vi "initialisationHWError.vi"(8 "error in (no error)":errorcluster, 11 "AtomChipHWC in":refnum<class "AtomChipHWC.lvclass">) -> (0 "error out":errorcluster, 3 "AtomChipHWC out":refnum<class "AtomChipHWC.lvclass">)   [LabVIEW 2009, in "Hardware.lvlib" / "HWControllers.lvlib" / "AtomChipHWC.lvclass"]
uses:
  AtomChipHWC.lvclass
  AtomChipHWC.lvclass/AtomChipHWC.ctl
  Channels/Digital/DigitalOutput.lvclass
  Channels/VoltOutput/AnalogOutput.lvclass
  Channels/DDSOutput/Generic/DDSOutput.lvclass
  Network Controllers/CameraNetworkController/CameraNetworkController.lvclass
  HWController.lvclass
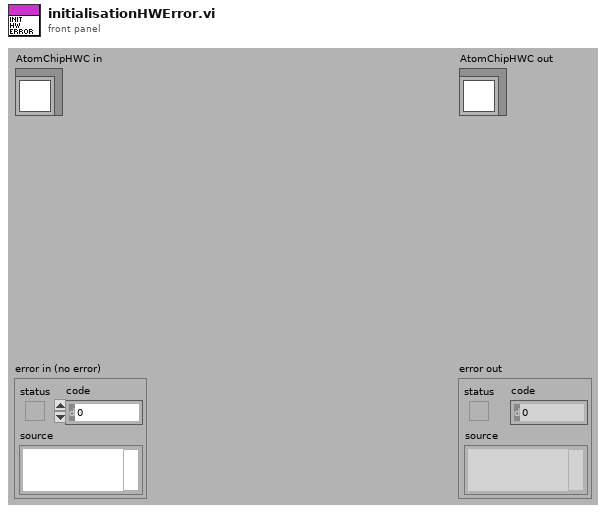
[diagram p1: front panel]
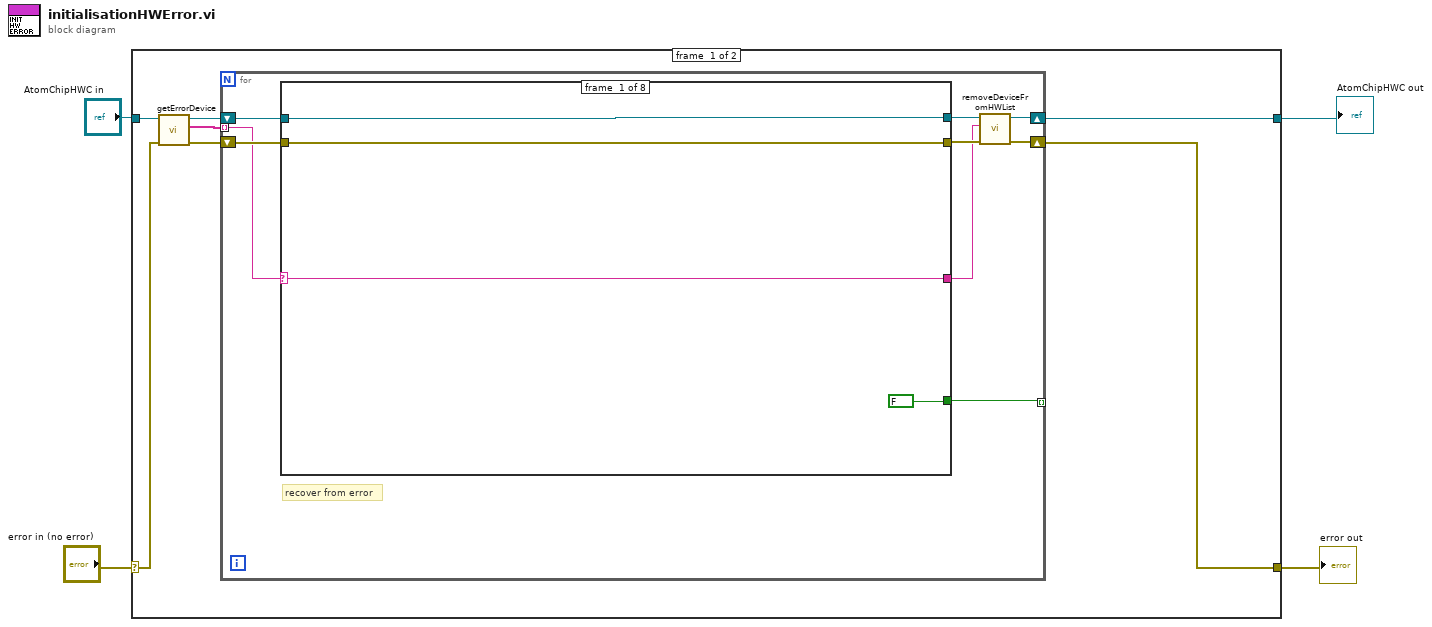
[diagram p0: block diagram]
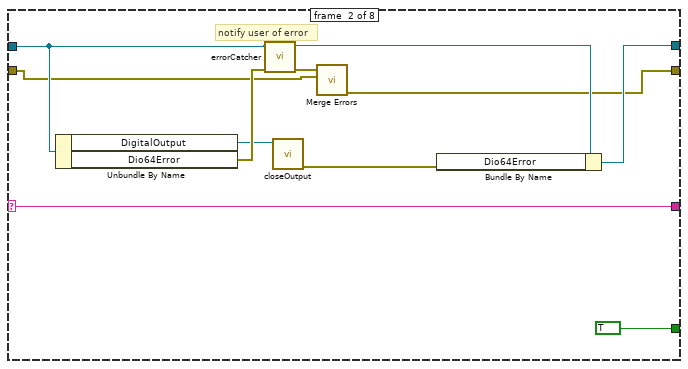
[diagram p2: hidden frame]
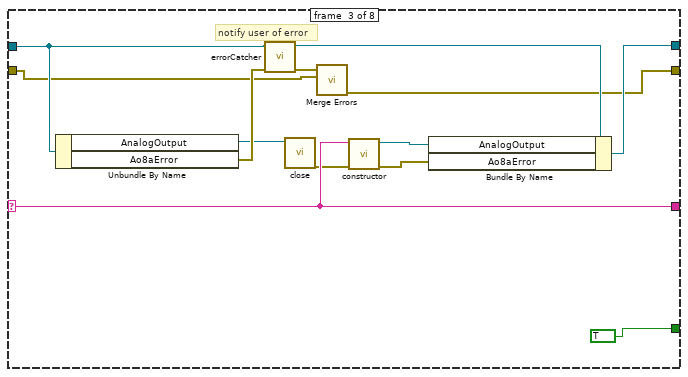
[diagram p3: hidden frame]
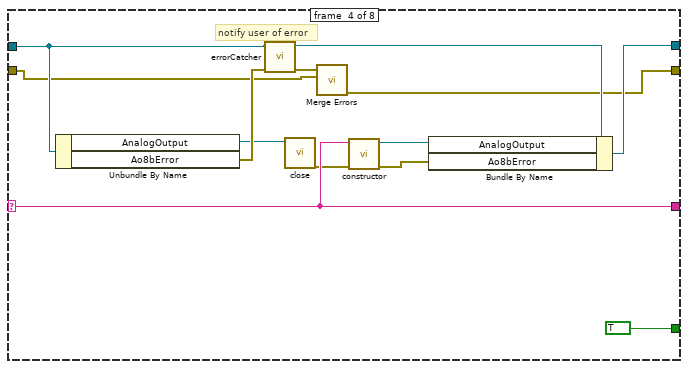
[diagram p4: hidden frame]
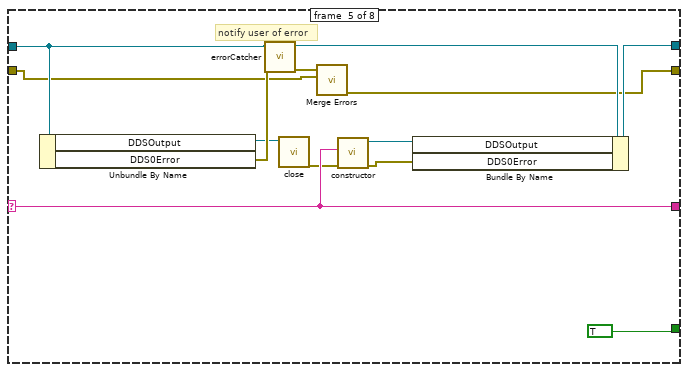
[diagram p5: hidden frame]
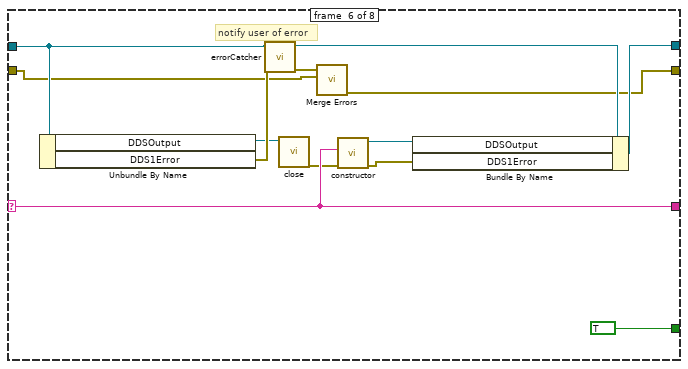
[diagram p6: hidden frame]
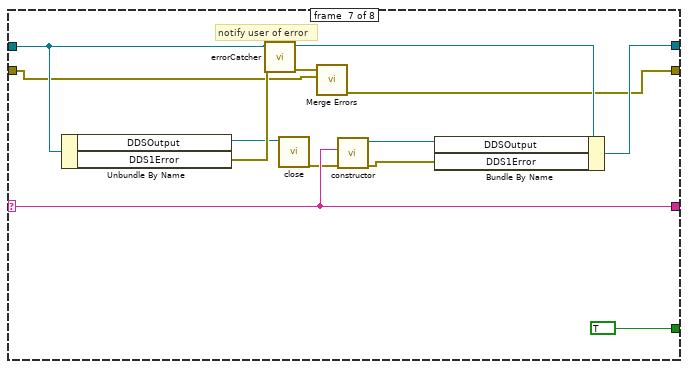
[diagram p7: hidden frame]
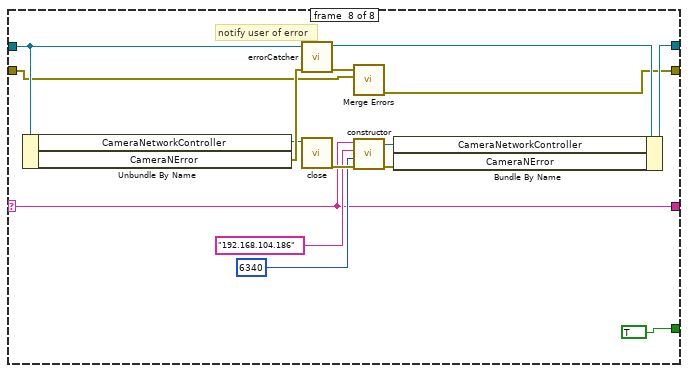
[diagram p8: hidden frame]
diagram:
  n1 = case shown="No Error" "error in (no error)" {
    selector: "error in (no error)" -> [w10 w116]
    tunnel: "AtomChipHWC in" -> [w11 w117]
    tunnel: [w6 w117] -> w2
    tunnel: [w5 w116] -> w1
    frame #0 {
      n2 = call "getErrorDevice.vi"("error in (no error)"=w10, "AtomChipHWC in"=w11) -> ("error out"=w7:errorcluster, "Devices"=w8:string[], "AtomChipHWC out"=w9:refnum<class "AtomChipHWC.lvclass">)  [unwired: 7 in]
      n3 = for {
        tunnel: w8 -> [w18] mode=indexing
        shift-right: [w14] -> w6
        shift-left: w9 -> [w20]
        shift-right: [w13] -> w5
        shift-left: w7 -> [w19]
        tunnel: [w12] -> _ mode=indexing
        # "recover from error"
        n4 = case shown="\"k3390\"" w18 {
          selector: w18 -> [w22 w28 w40 w53 w64 w77 w90 w102]
          tunnel: w20 -> [w24 w35 w48 w61 w74 w87 w100 w115]
          tunnel: [w24 w30 w43 w56 w69 w82 w95 w110] -> w17
          tunnel: [w23 w29 w42 w55 w68 w81 w94 w109] -> w16
          tunnel: w19 -> [w23 w31 w44 w57 w70 w83 w96 w111]
          tunnel: [w22 w28 w40 w53 w64 w77 w90 w102] -> w15
          tunnel: [FALSE TRUE TRUE TRUE TRUE TRUE TRUE TRUE] -> w12
          frame #0 {
          }
          frame #1 {
            # "notify user of error"
            n5 = Unbundle By Name(w35) -> ("DigitalOutput"=w26:refnum<class "DigitalOutput.lvclass">, "Dio64Error"=w33:errorcluster)
            n6 = call-dynamic "errorCatcher.vi"("error in (no error)"=w33, "HWController in"=w35) -> ("error out"=w32:errorcluster, "HWController out"=w34:refnum<class "AtomChipHWC.lvclass">)  [unwired: 8 in]
            n7 = call-dynamic "closeOutput.vi"("DigitalOutput in"=w26) -> ("error out"=w27:errorcluster)  [unwired: 10 in]
            n8 = call <vilib>:"Merge Errors.vi"("error in 2 (no error)"=w31, "error in 1 (no error)"=w32) -> ("error out"=w29:errorcluster)  [unwired: 5 in]
            n9 = Bundle By Name(cluster=w34, "Dio64Error"=w27) -> (w30:refnum<class "AtomChipHWC.lvclass">)
          }
          frame #2 {
            # "notify user of error"
            n10 = Unbundle By Name(w48) -> ("AnalogOutput"=w41:refnum<class "AnalogOutput.lvclass">, "Ao8aError"=w46:errorcluster)
            n11 = call-dynamic "errorCatcher.vi"("error in (no error)"=w46, "HWController in"=w48) -> ("error out"=w45:errorcluster, "HWController out"=w47:refnum<class "AtomChipHWC.lvclass">)  [unwired: 8 in]
            n12 = call-dynamic "close.vi"("AnalogOutput in"=w41) -> ("error out"=w39:errorcluster)  [unwired: 10 in]
            n13 = call <vilib>:"Merge Errors.vi"("error in 2 (no error)"=w44, "error in 1 (no error)"=w45) -> ("error out"=w42:errorcluster)  [unwired: 5 in]
            n14 = call "constructor.vi"("error in (no error)"=w39, "deviceName"=w40) -> ("error out"=w37:errorcluster, "AnalogOutput out"=w38:refnum<class "AnalogOutput.lvclass">)  [unwired: 8 in]
            n15 = Bundle By Name(cluster=w47, "AnalogOutput"=w38, "Ao8aError"=w37) -> (w43:refnum<class "AtomChipHWC.lvclass">)
          }
          frame #3 {
            # "notify user of error"
            n16 = Unbundle By Name(w61) -> ("AnalogOutput"=w54:refnum<class "AnalogOutput.lvclass">, "Ao8bError"=w59:errorcluster)
            n17 = call-dynamic "errorCatcher.vi"("error in (no error)"=w59, "HWController in"=w61) -> ("error out"=w58:errorcluster, "HWController out"=w60:refnum<class "AtomChipHWC.lvclass">)  [unwired: 8 in]
            n18 = call-dynamic "close.vi"("AnalogOutput in"=w54) -> ("error out"=w52:errorcluster)  [unwired: 10 in]
            n19 = call <vilib>:"Merge Errors.vi"("error in 2 (no error)"=w57, "error in 1 (no error)"=w58) -> ("error out"=w55:errorcluster)  [unwired: 5 in]
            n20 = call "constructor.vi"("error in (no error)"=w52, "deviceName"=w53) -> ("error out"=w50:errorcluster, "AnalogOutput out"=w51:refnum<class "AnalogOutput.lvclass">)  [unwired: 8 in]
            n21 = Bundle By Name(cluster=w60, "AnalogOutput"=w51, "Ao8bError"=w50) -> (w56:refnum<class "AtomChipHWC.lvclass">)
          }
          frame #4 {
            # "notify user of error"
            n22 = Unbundle By Name(w74) -> ("DDSOutput"=w67:refnum<class "DDSOutput.lvclass">, "DDS0Error"=w72:errorcluster)
            n23 = call-dynamic "errorCatcher.vi"("error in (no error)"=w72, "HWController in"=w74) -> ("error out"=w71:errorcluster, "HWController out"=w73:refnum<class "AtomChipHWC.lvclass">)  [unwired: 8 in]
            n24 = call-dynamic "close.vi"("DDSOutput in"=w67) -> ("error out"=w63:errorcluster)  [unwired: 10 in]
            n25 = call <vilib>:"Merge Errors.vi"("error in 2 (no error)"=w70, "error in 1 (no error)"=w71) -> ("error out"=w68:errorcluster)  [unwired: 5 in]
            n26 = call "constructor.vi"("error in (no error)"=w63, "device"=w64) -> ("error out"=w65:errorcluster, "DDSOutput out"=w66:refnum<class "DDSOutput.lvclass">)  [unwired: 8 in]
            n27 = Bundle By Name(cluster=w73, "DDSOutput"=w66, "DDS0Error"=w65) -> (w69:refnum<class "AtomChipHWC.lvclass">)
          }
          frame #5 {
            # "notify user of error"
            n28 = Unbundle By Name(w87) -> ("DDSOutput"=w80:refnum<class "DDSOutput.lvclass">, "DDS1Error"=w85:errorcluster)
            n29 = call-dynamic "errorCatcher.vi"("error in (no error)"=w85, "HWController in"=w87) -> ("error out"=w84:errorcluster, "HWController out"=w86:refnum<class "AtomChipHWC.lvclass">)  [unwired: 8 in]
            n30 = call-dynamic "close.vi"("DDSOutput in"=w80) -> ("error out"=w76:errorcluster)  [unwired: 10 in]
            n31 = call <vilib>:"Merge Errors.vi"("error in 2 (no error)"=w83, "error in 1 (no error)"=w84) -> ("error out"=w81:errorcluster)  [unwired: 5 in]
            n32 = call "constructor.vi"("error in (no error)"=w76, "device"=w77) -> ("error out"=w78:errorcluster, "DDSOutput out"=w79:refnum<class "DDSOutput.lvclass">)  [unwired: 8 in]
            n33 = Bundle By Name(cluster=w86, "DDSOutput"=w79, "DDS1Error"=w78) -> (w82:refnum<class "AtomChipHWC.lvclass">)
          }
          frame #6 {
            # "notify user of error"
            n34 = Unbundle By Name(w100) -> ("DDSOutput"=w93:refnum<class "DDSOutput.lvclass">, "DDS1Error"=w98:errorcluster)
            n35 = call-dynamic "errorCatcher.vi"("error in (no error)"=w98, "HWController in"=w100) -> ("error out"=w97:errorcluster, "HWController out"=w99:refnum<class "AtomChipHWC.lvclass">)  [unwired: 8 in]
            n36 = call-dynamic "close.vi"("DDSOutput in"=w93) -> ("error out"=w89:errorcluster)  [unwired: 10 in]
            n37 = call <vilib>:"Merge Errors.vi"("error in 2 (no error)"=w96, "error in 1 (no error)"=w97) -> ("error out"=w94:errorcluster)  [unwired: 5 in]
            n38 = call "constructor.vi"("error in (no error)"=w89, "device"=w90) -> ("error out"=w91:errorcluster, "DDSOutput out"=w92:refnum<class "DDSOutput.lvclass">)  [unwired: 8 in]
            n39 = Bundle By Name(cluster=w99, "DDSOutput"=w92, "DDS1Error"=w91) -> (w95:refnum<class "AtomChipHWC.lvclass">)
          }
          frame #7 {
            # "notify user of error"
            n40 = Unbundle By Name(w115) -> ("CameraNetworkController"=w108:refnum<class "CameraNetworkController.lvclass">, "CameraNError"=w113:errorcluster)
            n41 = call-dynamic "errorCatcher.vi"("error in (no error)"=w113, "HWController in"=w115) -> ("error out"=w112:errorcluster, "HWController out"=w114:refnum<class "AtomChipHWC.lvclass">)  [unwired: 8 in]
            n42 = call "close.vi"("CameraNetworkController in"=w108) -> ("error out"=w105:errorcluster)  [unwired: 9 in, 1 out]
            n43 = call <vilib>:"Merge Errors.vi"("error in 2 (no error)"=w111, "error in 1 (no error)"=w112) -> ("error out"=w109:errorcluster)  [unwired: 5 in]
            n44 = call "constructor.vi"("error in (no error)"=w105, "remote port"=u16 6340, "remote address"="192.168.104.186", "camera"=w102) -> ("error out"=w106:errorcluster, "CameraNetworkController out"=w107:refnum<class "CameraNetworkController.lvclass">)  [unwired: 6 in]
            n45 = Bundle By Name(cluster=w114, "CameraNetworkController"=w107, "CameraNError"=w106) -> (w110:refnum<class "AtomChipHWC.lvclass">)
          }
        }
        n46 = call "removeDeviceFromHWList.vi"("error in (no error)"=w16, "deviceName"=w15, "HWController in"=w17) -> ("error out"=w13:errorcluster, "HWController out"=w14:refnum<class "AtomChipHWC.lvclass">)  [unwired: 7 in]
      }
    }
    frame #1 {
    }
  }
  "error out" <- w1
  "AtomChipHWC out" <- w2
